vi "SpecificVI - Modals subVI Caller.vi"(11 "Sequence Context In":refnum<k7>) -> ()   [LabVIEW 2009]
uses:
  <vilib>/addons/TestStand/_TSUtility.llb/TestStand - End Modal Dialog (Sequence Context).vi
  <vilib>/addons/TestStand/_TSUtility.llb/TestStand - Start Modal Dialog (Sequence Context).vi
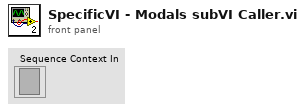
[diagram p1: front panel]
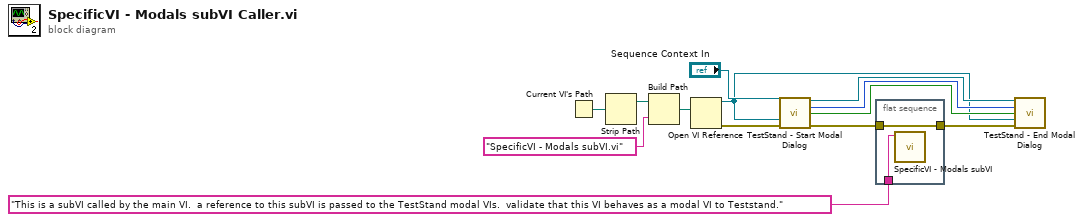
[diagram p0: block diagram]
diagram:
  n1 = Current VI's Path() -> (path=w13:path)
  n2 = Strip Path(path=w13) -> (stripped path=w12:path)  [unwired: 1 out]
  n3 = Build Path(base path=w12, name or relative path="SpecificVI - Modals subVI.vi") -> (appended path=w10:path)
  n4 = Open VI Reference(vi path=w10) -> (vi reference=w2:refnum<vi>, error out=w9:errorcluster)  [unwired: 5 in]
  n5 = call-poly <vilib>:"TestStand - Start Modal Dialog.vi"("Sequence Context In"="Sequence Context In", "VI to make Modal (Current VI)"=w2, "error in (no error)"=w9) -> ("Sequence Context Out"=w6:refnum<k7>, "Modal ID"=w4:i32, "VI Originally Open"=w3:bool, "error out"=w8:errorcluster)  [unwired: 8 in, 1 out]
  n6 = flat-sequence {
    tunnel: w8 -> [w15]
    tunnel: [w15] -> w7
    tunnel: "This is a subVI called by the main VI.  a reference to this subVI is passed to the TestStand modal VIs.  validate that this VI behaves as a modal VI to Teststand." ("name or relative path") -> [w14]
    frame #0 {
      n7 = call "SpecificVI - Modals subVI.vi"("Description"=w14) -> ()  [unwired: 11 in]
    }
  }
  n8 = call-poly <vilib>:"TestStand - End Modal Dialog.vi"("Sequence Context In"=w6, "Modal ID"=w4, "VI Originally Open"=w3, "VI to make non-Modal (Current VI)"=w2, "error in (no error)"=w7) -> ()  [unwired: 10 in, 1 out]
